vi "Steam Turbine Model.vi"(0 "Width (m)":i32=5 min=5 max=17 step=2, 1 "Height (m)":i32=5 min=4 max=9 step=1, 2 "Rotor Height":i32=1 min=0 max=1 step=1, 4 "Condensers":i32=5 max=8 step=1, 5 "Vents":i32=5 max=33 step=1) -> (10 "Energy Production (FE)":ext format="%.2f", 13 "Energy Production\nEfficiency (η)":ext, 14 "Flow (mB/t)":i64, 15 "Water Return (mB/t)":i64, 16 "Vents Limiting":bool, 17 "Dispersers Limiting":bool, 18 "Blades Limiting":bool, 19 "Coils Limiting":bool)   [LabVIEW 2023]
uses:
  Turbine Build Properties.ctl
  3be1dc29-0b19-cf4e-b19d-55a090115d5f.vi
  bbb8b91a-5175-7941-9f9e-431f1dc08699.vi
panel:
  out "Turbine Build Properties":T1 {"Energy Capacity (FE)" format="%.2f"}
  out "Max Condenser\nLayers":i32
  in  "Condenser\nLayers":i32=1 min=0 max=1 step=1
  out "Max Vents":i32 max=8
  out "Return Limited":bool
  out "Max Condensers":i32 max=8
  out "Maximum Height (m)":i32
  out "Maximum Rotor Height (m)":i32
  in  "Length (m)":i32=5 min=5 max=17 step=2
  # "Industrial Turbine Build"
  # "Industrial Turbine Properties"
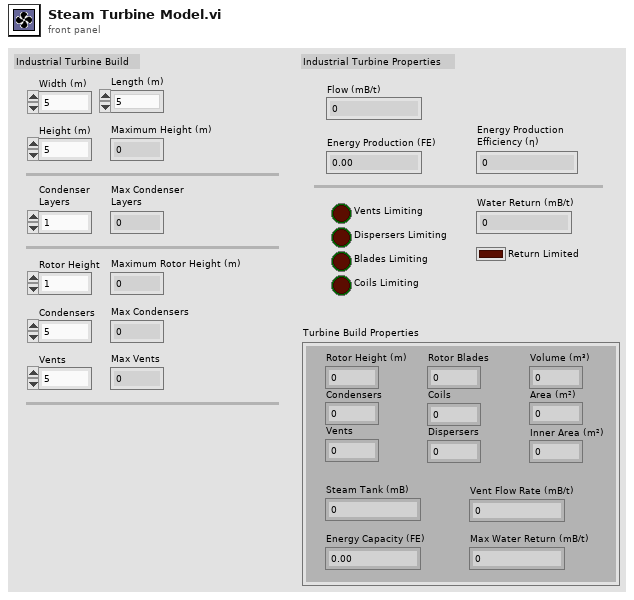
[diagram p1: front panel]
types:
  T1 = typedef "Turbine Build Properties.ctl" = cluster{"Volume (m³)":i32, "Rotor Height (m)":i32, "Condensers":i32, "Vents":i32, "Rotor Blades":i32, "Coils":i32, "Dispersers":i32, "Steam Tank (mB)":i64, "Energy Capacity (FE)":ext, "Vent Flow Rate (mB/t)":dbl, "Max Water Return (mB/t)":i32, "Area (m²)":i32, "Inner Area (m²)":i32}
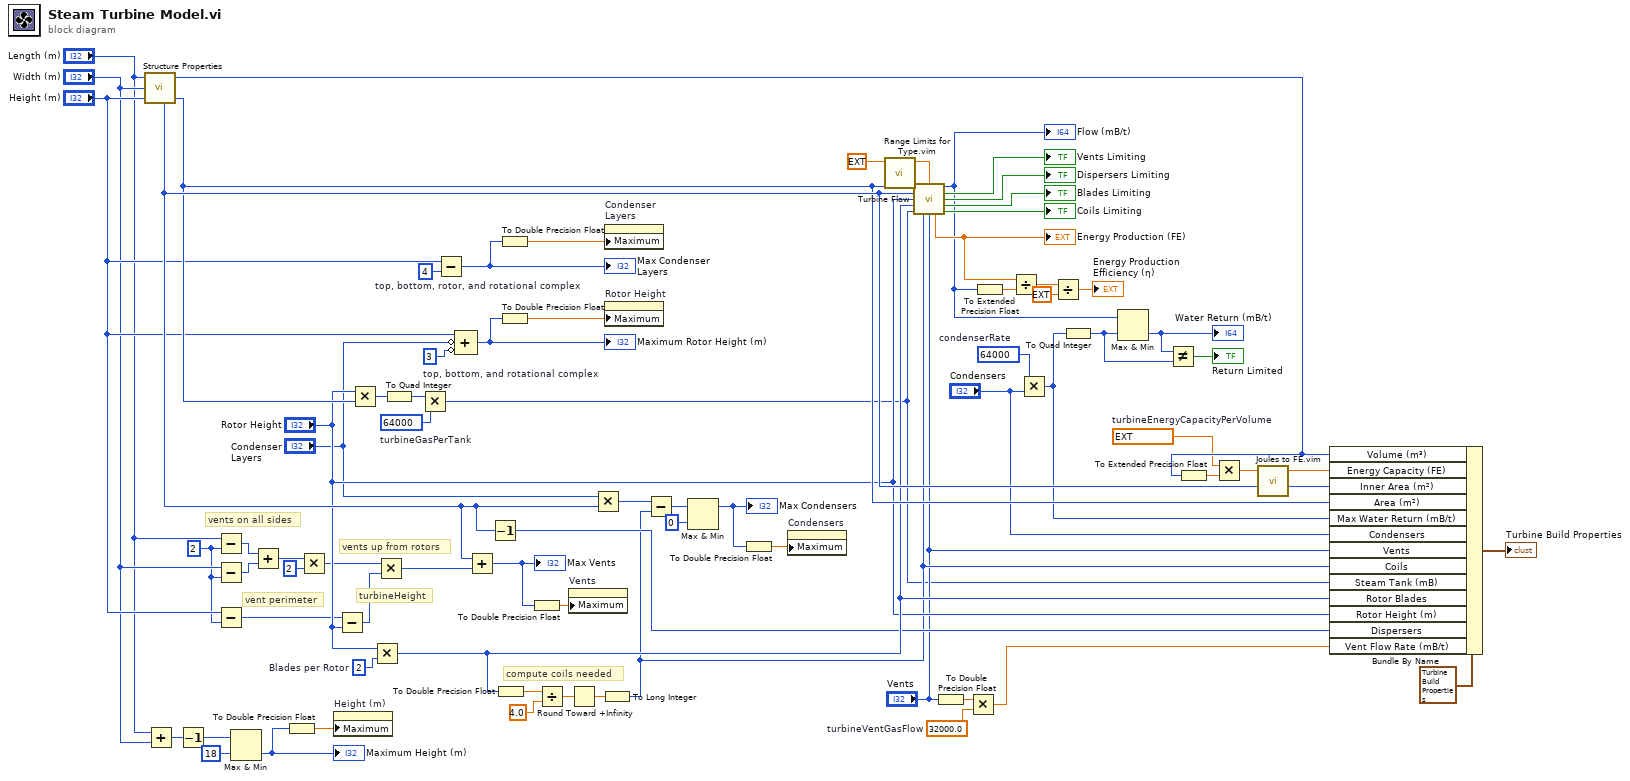
[diagram p0: block diagram]
diagram:
  w21 = 2 ("y")
  w27 = 4  # top, bottom, rotor, and rotational complex
  w1 = ext 16000000.0  # turbineEnergyCapacityPerVolume
  w29 = 3  # top, bottom, and rotational complex
  w52 = 64000  # condenserRate
  w57 = 32000.0  # turbineVentGasFlow
  w58 = 2  # Blades per Rotor
  w62 = i64 64000  # turbineGasPerTank
  # "compute coils needed"
  # "turbineHeight"
  # "vent perimeter"
  # "vents up from rotors"
  # "vents on all sides"
  n1 = call "Structure Properties.vi"("Length"="Length (m)", "Width"="Width (m)", "Height"="Height (m)") -> ("Volume"=w3:i32, "Inner Area"=w75:i32, "Area"=w74:i32)  [unwired: 2 in, 2 out]
  n2 = Add(x="Length (m)", y="Width (m)") -> (x+y=w31:i32)
  n3 = Decrement(x=w31) -> (x-1=w64:i32)
  n4 = Subtract(x="Length (m)", y=w21) -> (x-y=w20:i32)
  n5 = Subtract(x="Width (m)", y=w21) -> (x-y=w19:i32)
  n6 = Subtract(x="Height (m)", y=w21) -> (x-y=w40:i32)
  n7 = Max & Min(x=w64, y=18) -> (min(x,y)=w61:i32)  [unwired: 1 out]
  "Maximum Height (m)" <- w61
  n8 = Add(x=w20, y=w19) -> (x+y=w18:i32)
  n9 = To Double Precision Float(number=w61) -> (double precision float=w60:dbl)
  n10 = Multiply(x=w18, y=2) -> (x*y=w16:i32)
  n11 = property on="Height (m)" class="DigNum (strict)"("Maximum"=w60) -> ()  [unwired: 2 in, 2 out]
  n12 = Subtract(x=w40, y="Rotor Height") -> (x-y=w42:i32)
  n13 = Multiply(x="Rotor Height", y=w74) -> (x*y=w63:i32)
  n14 = Multiply(x="Rotor Height", y=w58) -> (x*y=w73:i32)
  n15 = Multiply(x=w16, y=w42) -> (x*y=w14:i32)
  n16 = To Quad Integer(1:w63) -> (0:w23:i64)
  n17 = Multiply(x=w23, y=w62) -> (x*y=w4:i64)
  n18 = Subtract(x="Height (m)", y=w27) -> (x-y=w28:i32)
  "Max Condenser\nLayers" <- w28
  n19 = Compound Arithmetic op=ADD("Height (m)", invert "Condenser\nLayers", invert w29) -> (w30:i32)
  "Maximum Rotor Height (m)" <- w30
  n20 = Add(x=w75, y=w14) -> (x+y=w10:i32)
  "Max Vents" <- w10
  n21 = Decrement(x=w75) -> (x-1=w72:i32)
  n22 = To Double Precision Float(number=w73) -> (double precision float=w56:dbl)
  n23 = To Double Precision Float(number=w28) -> (double precision float=w26:dbl)
  n24 = To Double Precision Float(number=w30) -> (double precision float=w59:dbl)
  n25 = To Double Precision Float(number=w10) -> (double precision float=w41:dbl)
  n26 = Divide(x=w56, y=4.0) -> (x/y=w54:dbl)
  n27 = property on="Vents" class="DigNum (strict)"("Maximum"=w41) -> ()  [unwired: 2 in, 2 out]
  n28 = Round Toward +Infinity(x=w54) -> (ceil(x): smallest int >= x=w53:dbl)
  n29 = Multiply(x="Condenser\nLayers", y=w75) -> (x*y=w22:i32)
  n30 = To Long Integer(number=w53) -> (32bit integer=w70:i32)
  n31 = property on="Condenser\nLayers" class="DigNum (strict)"("Maximum"=w26) -> ()  [unwired: 2 in, 2 out]
  n32 = property on="Rotor Height" class="DigNum (strict)"("Maximum"=w59) -> ()  [unwired: 2 in, 2 out]
  n33 = Subtract(x=w22, y=w70) -> (x-y=w12:i32)
  n34 = Max & Min(x=w12, y=0) -> (max(x,y)=w11:i32)  [unwired: 1 out]
  "Max Condensers" <- w11
  n35 = To Double Precision Float(number=w11) -> (double precision float=w51:dbl)
  n36 = property on="Condensers" class="DigNum (strict)"("Maximum"=w51) -> ()  [unwired: 2 in, 2 out]
  n37 = call "Range Limits for Type.vim"("type"=ext 0.0 ("Energy Needed (FE)")) -> ("maximum value for type"=w49:ext)  [unwired: 9 in, 1 out]
  n38 = call "Turbine Flow.vi"("Structure Area (m²)"=w74, "Energy Needed (FE)"=w49, "Inner Area (m²)"=w75, "Rotor Height (m)"="Rotor Height", "Blades"=w73, "Stored Gas (mB/t)"=w4, "Coils"=w70, "Vents"="Vents") -> ("Flow (mB/t)"=w39:i64, "Vents Limiting"=→"Vents Limiting":bool, "Dispersers Limiting"=→"Dispersers Limiting":bool, "Blades Limiting"=→"Blades Limiting":bool, "Energy Production (FE)"=w68:ext, "Coils Limiting"=→"Coils Limiting":bool)  [unwired: 1 in, 1 out]
  "Energy Production (FE)" <- w68
  "Flow (mB/t)" <- w39
  n39 = To Double Precision Float(number="Vents") -> (double precision float=w24:dbl)
  n40 = Multiply(x=w24, y=w57) -> (x*y=w5:dbl)
  n41 = To Extended Precision Float(1:w39) -> (0:w38:ext)
  n42 = Divide(x=w68, y=w38) -> (x/y=w37:ext)
  n43 = Multiply(x=w52, y="Condensers") -> (x*y=w7:i32)
  n44 = Divide(x=w37, y=ext 4.0) -> (x/y=→"Energy Production\nEfficiency (η)":ext)
  n45 = To Quad Integer(1:w7) -> (0:w25:i64)
  n46 = Max & Min(x=w39, y=w25) -> (min(x,y)=w44:i64)  [unwired: 1 out]
  "Water Return (mB/t)" <- w44
  n47 = Not Equal?(x=w44, y=w25) -> (x != y?=→"Return Limited":bool)
  n48 = To Extended Precision Float(1:w3) -> (0:w33:ext)
  n49 = Multiply(x=w1, y=w33) -> (x*y=w34:ext)
  n50 = call "Joules to FE.vim"("J"=w34) -> ("FE"=w2:ext)  [unwired: 4 in]
  n51 = Bundle By Name(cluster=T1 {"Volume (m³)"=0, "Rotor Height (m)"=0, "Condensers"=0, "Vents"=0, "Rotor Blades"=0, "Coils"=0, "Dispersers"=0, "Steam Tank (mB)"=0, "Energy Capacity (FE)"=0.0, "Vent Flow Rate (mB/t)"=0.0, "Max Water Return (mB/t)"=0, "Area (m²)"=0, "Inner Area (m²)"=0} ("Turbine Build Properties"), "Volume (m³)"=w3, "Energy Capacity (FE)"=w2, "Inner Area (m²)"=w75, "Area (m²)"=w74, "Max Water Return (mB/t)"=w7, "Condensers"="Condensers", "Vents"="Vents", "Coils"=w70, "Steam Tank (mB)"=w4, "Rotor Blades"=w73, "Rotor Height (m)"="Rotor Height", "Dispersers"=w72, "Vent Flow Rate (mB/t)"=w5) -> (→"Turbine Build Properties":T1)
